vi "niDTS Template RF Test Initialize.vi"(0 "Dut Reference":T2, 5 "SystemTechnologyCatalog":refnum<class "niDTS SystemTechnologyCatalog.lvclass">, 7 "SystemDut":refnum<class "niDTS SystemDut.lvclass">, 9 "Logger Reference":T1, 11 "error in (no error)":errorcluster) -> (4 "Template Tx Test Handle":T3, 6 "AllowAsync":bool=TRUE, 15 "error out":errorcluster)   [LabVIEW 2014, in "niDTS Template.lvlib"]
uses:
  niDTS Template.lvlib
  Includes/Template RF Test INC Handle.ctl
  Objects/BASE_class/Template RF Test.lvclass
  Framework/Dut/Includes/niDTS Dut INC Handle.ctl
  Framework/Dut/Objects/BASE_class/niDTS Dut.lvclass
  Framework/Logger/Includes/niDTS Logger INC Handle.ctl
  Framework/Logger/Objects/BASE_class/niDTS Logger.lvclass
  TestStand/Station/Objects/SystemTechnologyCatalog/niDTS SystemTechnologyCatalog.lvclass
  TestStand/Station/Objects/SystemDut/niDTS SystemDut.lvclass
  TestStand/niDTS TestStand.lvlib
  Framework/niDTS Framework.lvlib
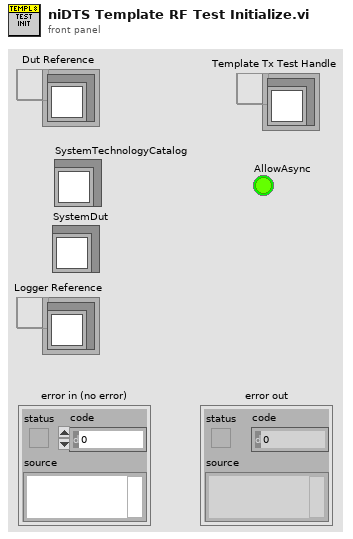
[diagram p1: front panel]
types:
  T1 = typedef "niDTS Framework.lvlib/niDTS Logger INC Handle.ctl" = refnum<data-value>
  T2 = typedef "niDTS Framework.lvlib/niDTS Dut INC Handle.ctl" = refnum<data-value>
  T3 = typedef "niDTS Template.lvlib/Template RF Test INC Handle.ctl" = refnum<data-value>
  T4 = typedef "niDTS TestStand.lvlib/niDTS TestStep INC Handle.ctl" = refnum<data-value>
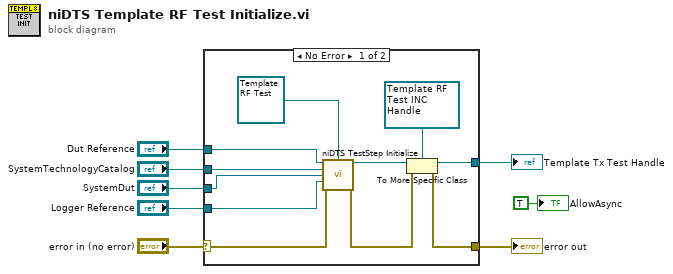
[diagram p0: block diagram]
diagram:
  n1 = case shown="No Error" "error in (no error)" {
    selector: "error in (no error)" -> [w16 w20]
    tunnel: [w17 w20] -> w8
    tunnel: [w15 _] -> w6
    tunnel: "Dut Reference" -> [w12 _]
    tunnel: "SystemTechnologyCatalog" -> [w11 _]
    tunnel: "SystemDut" -> [w10 _]
    tunnel: "Logger Reference" -> [w9 _]
    frame No Error {
      n2 = call "niDTS TestStep Initialize.vi"("Dut Handle"=w12, "Test Type"=refnum<class "Template RF Test.lvclass"> refnum ("Template.lvlib:Template Tx Test.lvclass"), "SystemTechnologyCatalog"=w11, "SystemDut"=w10, "Logger Reference"=w9, "error in (no error)"=w16) -> ("Test Handle out"=w19:T4, "error out"=w18:errorcluster)  [unwired: 8 in]
      n3 = To More Specific Class(target class=T3 refnum ("Template Tx Test Handle"), reference=w19, error in=w18) -> (specific class reference=w15:T3, error out=w17:errorcluster)
    }
    frame Error {
    }
  }
  "error out" <- w8
  "Template Tx Test Handle" <- w6
  "AllowAsync" <- TRUE ("AllowAsync")
